vi "Main.vi"() -> ()   [LabVIEW 2020, in "Hardware Abstraction App.lvclass"]
uses:
  Hardware Abstraction App/Hardware Abstraction App.lvclass
  Devices/PLC/PLC.lvclass
  C:/Users/fflores/Documents/GitHub Projects/OOP-Concepts-in-LabVIEW/Pillars of OOD/Hardware Abstraction/Devices/AutomatedController/AutomatedController.lvclass
  Devices/OPC/OPC.lvclass
  Devices/cRIO/cRIO.lvclass
  Devices/Arduino/Arduino.lvclass
  Devices/AutomatedController/AutomatedController.lvclass
panel:
  in  "Stop Button":bool
  in  "Dispositivo":i32(listbox)=3
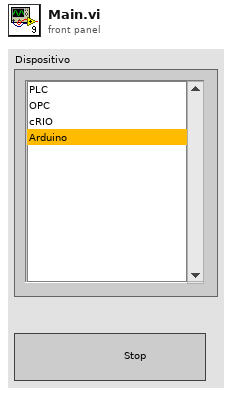
[diagram p1: front panel]
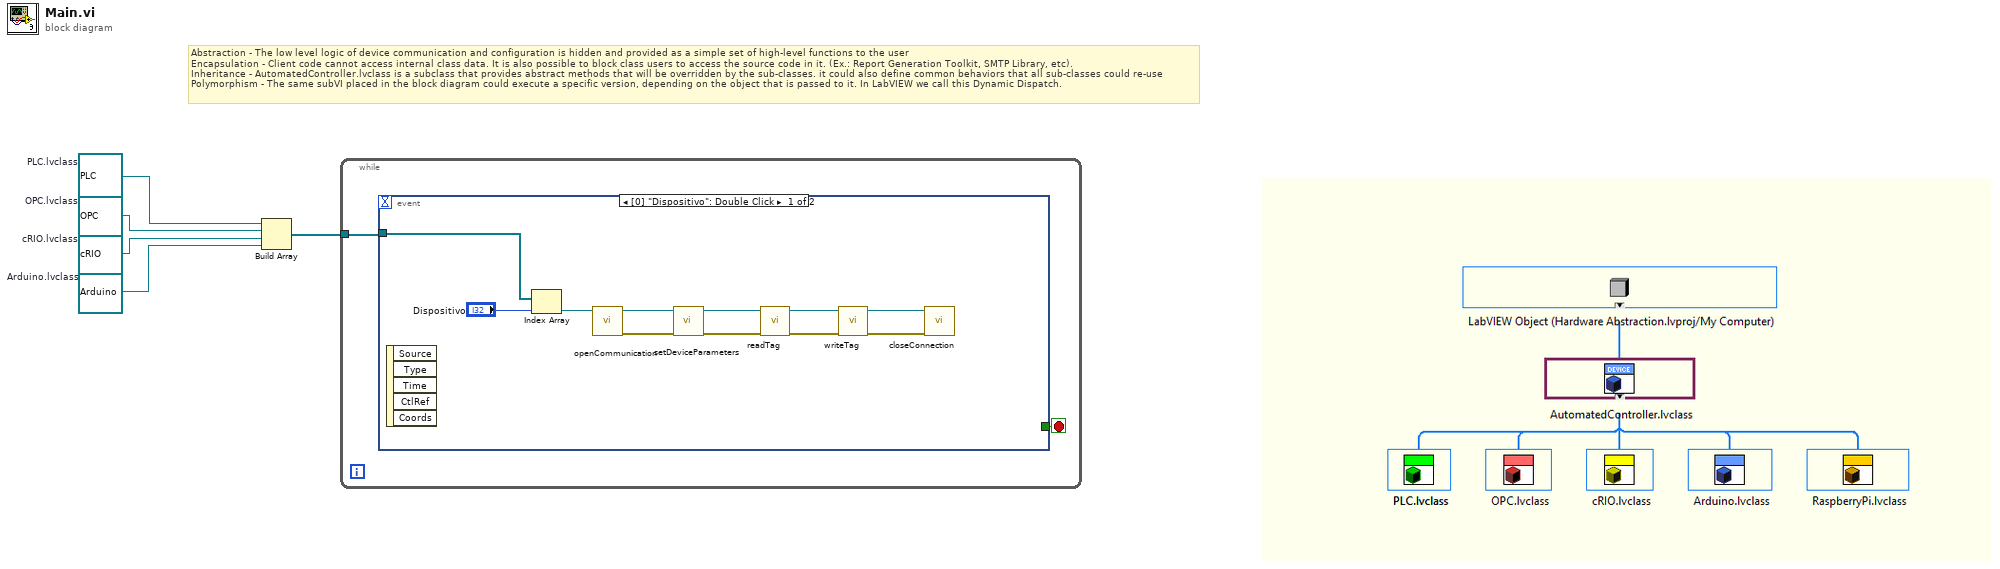
[diagram p0: block diagram]
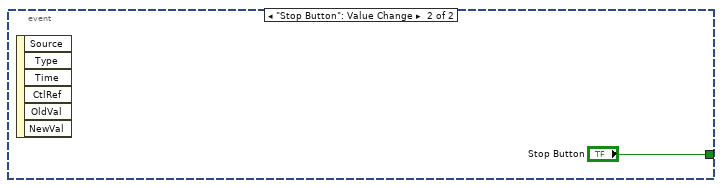
[diagram p2: hidden frame]
diagram:
  w2 = refnum<class "Arduino.lvclass"> refnum  # Arduino.lvclass
  w3 = refnum<class "cRIO.lvclass"> refnum  # cRIO.lvclass
  w4 = refnum<class "OPC.lvclass"> refnum  # OPC.lvclass
  w5 = refnum<class "PLC.lvclass"> refnum  # PLC.lvclass
  # "Abstraction - The low level logic of device communication and configuration is hidden and provided as a simple set of high-level functions to the user\nEncapsulation - Client code cannot access internal class data. It is also possible to block class users to access the source code in it. (Ex.: Report Generation Toolkit, SMTP Library, etc).\nInheritance - AutomatedController.lvclass is a subclass that provides abstract methods that will be overridden by the sub-classes. it could also define common behaviors that all sub-classes could re-use\nPolymorphism - The same subVI placed in the block diagram could execute a specific version, depending on the object that is passed to it. In LabVIEW we call this Dynamic Dispatch."
  n1 = Build Array(w5, w4, w3, w2) -> (w1:refnum<class "AutomatedController.lvclass">[])
  n2 = while {
    tunnel: w1 -> [w6]
    stop <- w7 stop-if-true
    n3 = event shown="[0] \"Dispositivo\": Double Click" {
      selector: _ -> [_ _]
      dyn-events: _ -> [_ _]
      timeout: _ -> [_ _]
      tunnel: [_ "Stop Button"] -> w7
      tunnel: w6 -> [w11 _]
      event "Dispositivo": Double Click {
        n4 = event-data() -> ()  [unwired: 1 in, 5 out]
        n5 = Index Array(array=w11, index="Dispositivo") -> (element=w9:refnum<class "AutomatedController.lvclass">)
        n6 = call-dynamic "openCommunication.vi"("AutomatedController in"=w9) -> ("error out"=w17:errorcluster, "AutomatedController out"=w18:refnum<class "AutomatedController.lvclass">)  [unwired: 9 in]
        n7 = call-dynamic "setDeviceParameters.vi"("error in (no error)"=w17, "AutomatedController in"=w18) -> ("error out"=w16:errorcluster, "AutomatedController out"=w8:refnum<class "AutomatedController.lvclass">)  [unwired: 8 in]
        n8 = call-dynamic "readTag.vi"("error in (no error)"=w16, "AutomatedController in"=w8) -> ("error out"=w14:errorcluster, "AutomatedController out"=w15:refnum<class "AutomatedController.lvclass">)  [unwired: 8 in]
        n9 = call-dynamic "writeTag.vi"("error in (no error)"=w14, "AutomatedController in"=w15) -> ("error out"=w12:errorcluster, "AutomatedController out"=w13:refnum<class "AutomatedController.lvclass">)  [unwired: 8 in]
        n10 = call-dynamic "closeConnection.vi"("error in (no error)"=w12, "AutomatedController in"=w13) -> ()  [unwired: 8 in, 2 out]
      }
      event "Stop Button": Value Change {
        n11 = event-data() -> ()  [unwired: 1 in, 6 out]
      }
    }
  }
